vi "Create Redirect Response.vi"   [LabVIEW 2020]
uses:
  <vilib>/IlluminatedG/IG HTTP Utils/HTTP Utils/Redirect Response/Redirect Response.lvclass
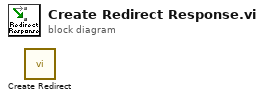
[diagram p0: block diagram]
diagram:
  n1 = call <vilib>:"Create Redirect.vi"() -> ()  [unwired: 10 in, 2 out]
